vi "2. ControlRealTimeEx2.vi"() -> ()   [LabVIEW 2011]
panel:
  out "Now":string[][](array[string])
  out "Forecast 2":string[][](array[string])
  out "Forecast 1":string[][](array[string])
  in  "IP Address":string(combo)="130.237.50.30"
  in  "Password":string
  in  "Username":string
  out "Access to HVAC Msg":errorcluster={"status"=FALSE, "code"=0, "source"="Please Wait ..."}
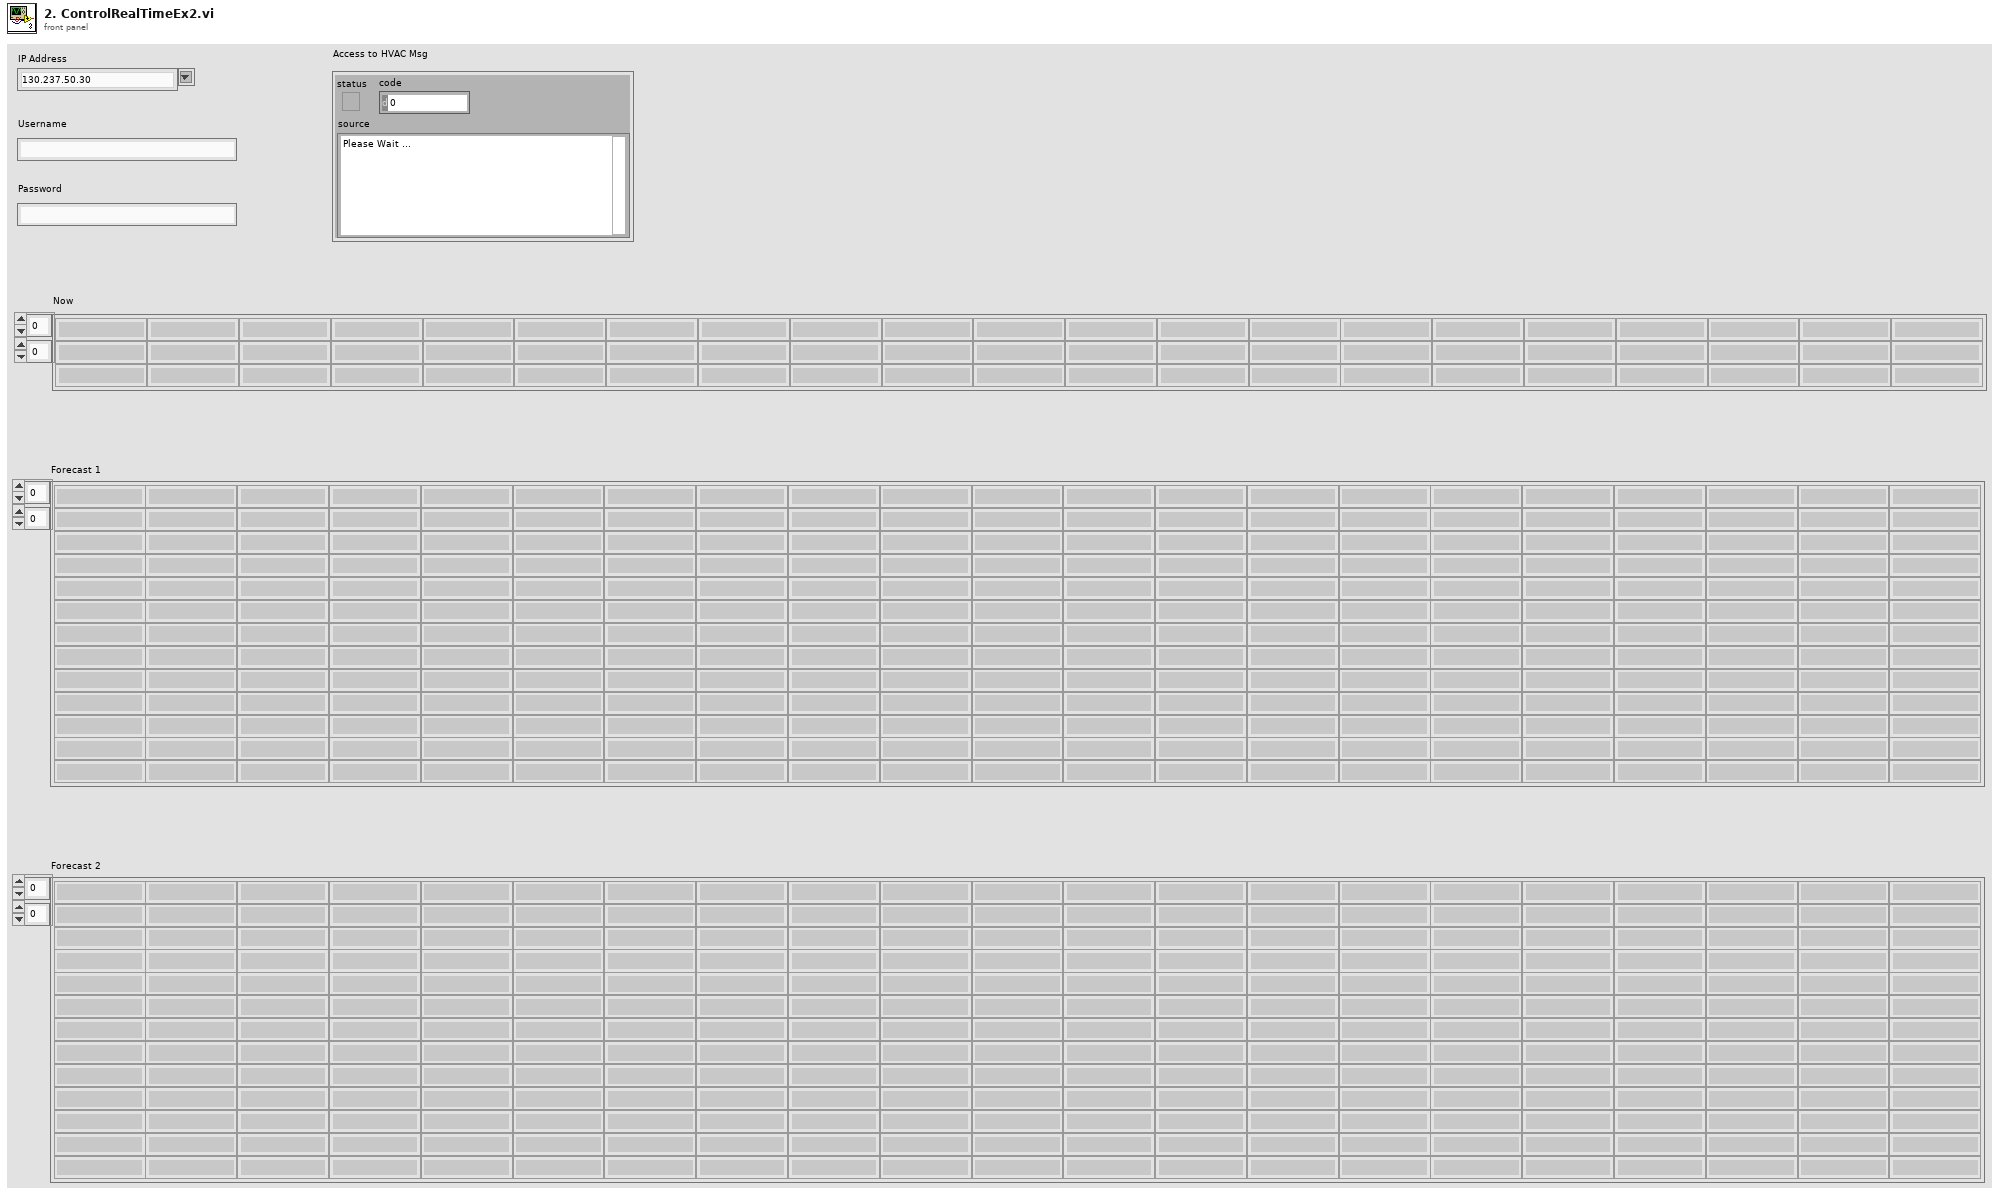
[diagram p1: front panel]
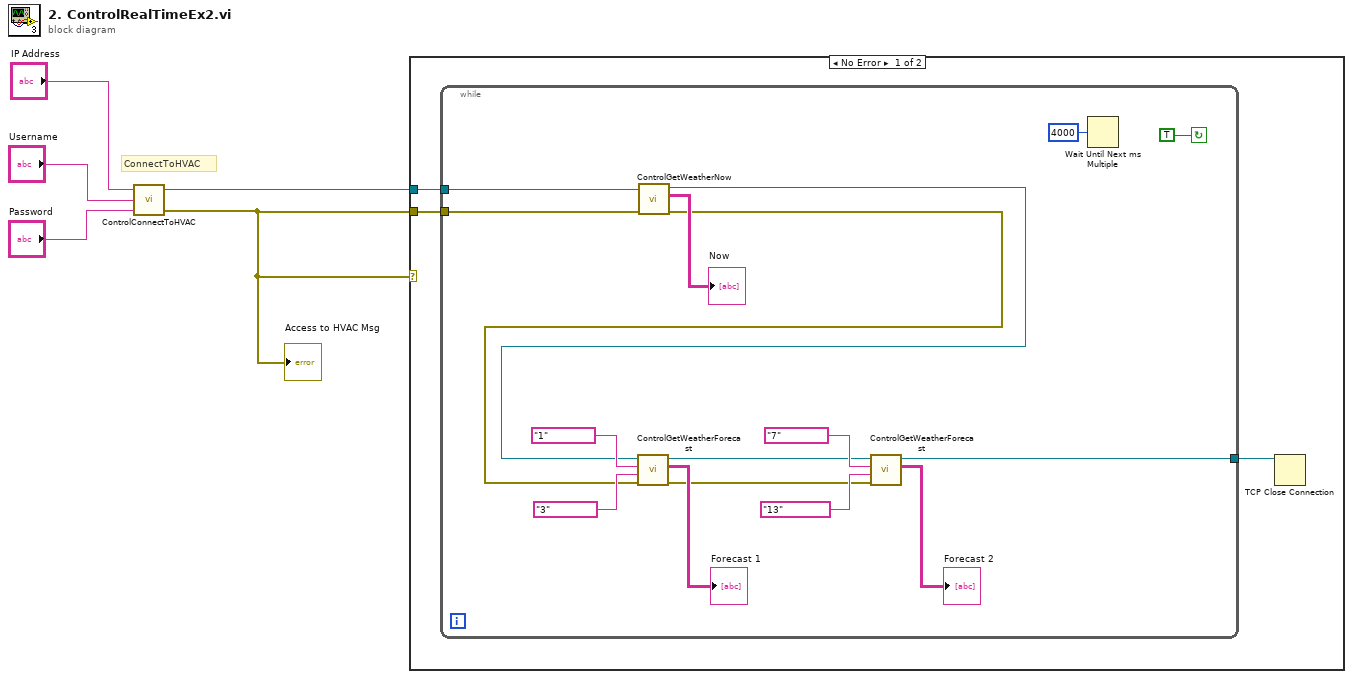
[diagram p0: block diagram]
diagram:
  # "ConnectToHVAC"
  n1 = call "ControlConnectToHVAC.vi"("Password"="Password", "Username"="Username", "IP Address"="IP Address") -> ("error out"=w4:errorcluster, "connection ID out"=w5:refnum<k5>)  [unwired: 1 in]
  "Access to HVAC Msg" <- w4
  n2 = case shown="No Error" w4 {
    tunnel: w5 -> [w8 _]
    tunnel: w4 -> [w7 _]
    frame No Error {
      n3 = while {
        tunnel: w8 -> [w13]
        tunnel: w7 -> [w12]
        tunnel: [w15] -> w6
        stop <- TRUE continue-if-true
        n4 = call "ControlGetWeatherNow.vi"("error in"=w12, "connection ID in"=w13) -> ("error out"=w9:errorcluster, "output array"=→"Now":string[][], "connection ID out"=w10:refnum<k5>)  [unwired: 6 in]
        n5 = call "ControlGetWeatherForecast.vi"("error in"=w9, "To"="3", "From"="1", "connection ID in"=w10) -> ("error out"=w17:errorcluster, "output array"=→"Forecast 1":string[][], "connection ID out"=w16:refnum<k5>)  [unwired: 4 in]
        n6 = call "ControlGetWeatherForecast.vi"("error in"=w17, "To"="13", "From"="7", "connection ID in"=w16) -> ("output array"=→"Forecast 2":string[][], "connection ID out"=w15:refnum<k5>)  [unwired: 4 in, 1 out]
        n7 = Wait Until Next ms Multiple(millisecond multiple=u32 4000) -> ()  [unwired: 1 out]
      }
      n8 = TCP Close Connection(connection ID=w6) -> ()  [unwired: 2 in, 2 out]
    }
    frame Error {
    }
  }
